vi "lvEtherbone.sdb_extract_device_info.vi"(2 "sdb_device_bin":u8[](array[numeric])) -> (12 "record_type":u8 format="%.0x", 13 "name":string, 14 "addr_first":u64 format="%.0x", 15 "addr_last":u64 format="%.0x", 16 "vendor_id":u64 format="%.0x", 17 "device_id":u32 format="%.0x", 18 "version":u32 format="%.0x", 19 "date":u32 format="%.0x")   [LabVIEW 2012, in "lvEtherbone.lvlib"]
uses:
  lvEtherbone.lvlib
panel:
  out "size(s)":i32
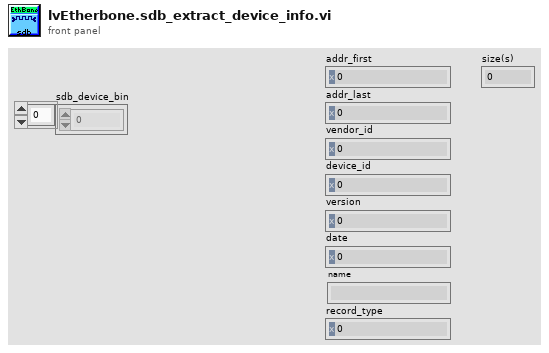
[diagram p1: front panel]
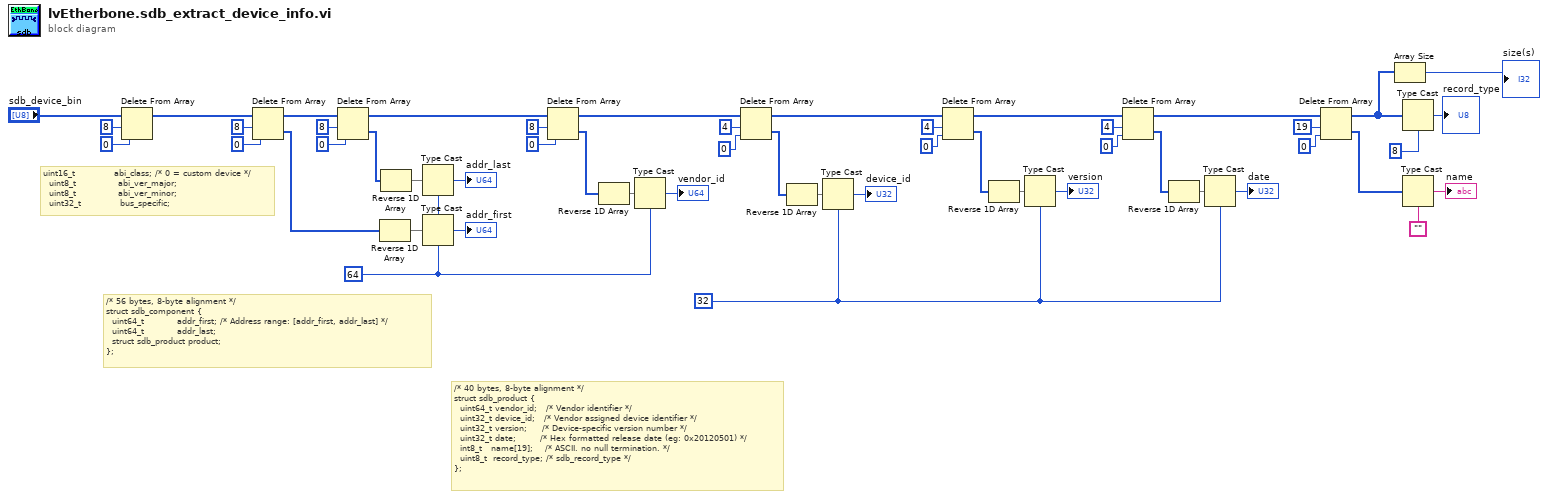
[diagram p0: block diagram]
diagram:
  w11 = u32 32 ("length")
  w35 = u64 64 ("length")
  # "/* 40 bytes, 8-byte alignment */\nstruct sdb_product {\n  uint64_t vendor_id;   /* Vendor identifier */\n  uint32_t device_id;   /* Vendor assigned device identifier */\n  uint32_t version;     /* Device-specific version number */\n  uint32_t date;        /* Hex formatted release date (eg: 0x20120501) */\n  int8_t   name[19];    /* ASCII. no null termination. */\n  uint8_t  record_type; /* sdb_record_type */\n};"
  # "/* 56 bytes, 8-byte alignment */\nstruct sdb_component {\n  uint64_t           addr_first; /* Address range: [addr_first, addr_last] */\n  uint64_t           addr_last;\n  struct sdb_product product;\n};"
  # "uint16_t             abi_class; /* 0 = custom device */\n  uint8_t              abi_ver_major;\n  uint8_t              abi_ver_minor;\n  uint32_t             bus_specific;"
  n1 = Delete From Array(array="sdb_device_bin", length=8, index=0) -> (array with subset deleted=w48:u8[])  [unwired: 1 out]
  n2 = Delete From Array(array=w48, length=8, index=0) -> (deleted portion=w47:u8[], array with subset deleted=w45:u8[])
  n3 = Delete From Array(array=w45, length=8, index=0) -> (deleted portion=w44:u8[], array with subset deleted=w38:u8[])
  n4 = Reverse 1D Array(array=w47) -> (reversed array=w32:u8[])
  n5 = Reverse 1D Array(array=w44) -> (reversed array=w34:u8[])
  n6 = Type Cast(type=w35, x=w34) -> (*(type *) &x=→"addr_last":u64)
  n7 = Type Cast(type=w35, x=w32) -> (*(type *) &x=→"addr_first":u64)
  n8 = Delete From Array(array=w38, length=8, index=0) -> (deleted portion=w36:u8[], array with subset deleted=w30:u8[])
  n9 = Reverse 1D Array(array=w36) -> (reversed array=w31:u8[])
  n10 = Type Cast(type=w35, x=w31) -> (*(type *) &x=→"vendor_id":u64)
  n11 = Delete From Array(array=w30, length=4, index=0) -> (deleted portion=w24:u8[], array with subset deleted=w18:u8[])
  n12 = Reverse 1D Array(array=w24) -> (reversed array=w26:u8[])
  n13 = Type Cast(type=w11, x=w26) -> (*(type *) &x=→"device_id":u32)
  n14 = Delete From Array(array=w18, length=4, index=0) -> (deleted portion=w23:u8[], array with subset deleted=w12:u8[])
  n15 = Reverse 1D Array(array=w23) -> (reversed array=w21:u8[])
  n16 = Type Cast(type=w11, x=w21) -> (*(type *) &x=→"version":u32)
  n17 = Delete From Array(array=w12, length=4, index=0) -> (deleted portion=w13:u8[], array with subset deleted=w7:u8[])
  n18 = Reverse 1D Array(array=w13) -> (reversed array=w15:u8[])
  n19 = Type Cast(type=w11, x=w15) -> (*(type *) &x=→"date":u32)
  n20 = Delete From Array(array=w7, length=19, index=0) -> (deleted portion=w5:u8[], array with subset deleted=w2:u8[])
  n21 = Array Size(array=w2) -> (size(s)=→"size(s)":i32)
  n22 = Type Cast(type=u8 8 ("length"), x=w2) -> (*(type *) &x=→"record_type":u8)
  n23 = Type Cast(type="", x=w5) -> (*(type *) &x=→"name":string)
